vi "Finish.vi"   [LabVIEW 2015]
doc: "This VI is called just before exiting. It is expected to close I/O refnum, save collected data, etc."
uses:
  <vilib>/Rock Robotics/WPI/Utilities/WPI_GetSetVariantRefNum.vi
types:
  T1 = typedef "WPI_RobotDriveDevRef.ctl" = cluster{"DevStatus":errorcluster, "Motors[]":T2[], "Square Inputs":bool, "Max Output":dbl}
  T2 = typedef "WPI_MotorControlDeviceRef.ctl" = cluster{"DeviceStatus":errorcluster, "Type":T3, "PWM":cluster{"PWM Channel":T4, "DeadBand":T5}, "CAN":cluster{"Device Number":u8, "Control Mode":T6, "Semaphore":T7, "Max Vout":dbl, "TalonSRX Control Mode":T8}, "Invert":bool}
  T3 = typedef "WPI_MotorControlType.ctl" = enum16{"PWM", "CAN", "CANTalonSRX"}
  T4 = typedef "FPGA_DIOPWMChannel.ctl" = enum8{"PWM 0", "PWM 1", "PWM 2", "PWM 3", "PWM 4", "PWM 5", "PWM 6", "PWM 7", "PWM 8", "PWM 9", "PWM MXP 0", "PWM MXP 1", "PWM MXP 2", "PWM MXP 3", "PWM MXP 4", "PWM MXP 5", "PWM MXP 6", "PWM MXP 7", "PWM MXP 8", "PWM MXP 9", "Invalid"}
  T5 = typedef "WPI_PWMDeadband.ctl" = cluster{"Name":string, "maxPositivePwm":i32, "minPositivePwm":i32, "centerPwm":i32, "maxNegativePwm":i32, "minNegativePwm":i32, "angularRange":u16}
  T6 = typedef "WPI_CANJaguar_ControlMode.ctl" = enum8{"Percent VBus", "Current", "Speed", "Position", "Voltage"}
  T7 = typedef "Semaphore RefNum" = refnum<k1>
  T8 = typedef "WPI_CANTalonSRX_APIControlMode.ctl" = enum8{"Percent VBus", "Speed", "Position", "Slave", "Unchanged / Invalid", "Voltage Compensation", "Current", "Motion Profile"}
  T9 = typedef "WPI_SerialPortRef.ctl" = cluster{"DevStatus":errorcluster, "Serial Port Name":refnum<visa-resource-name>}
  T10 = typedef "WPI_SolenoidDevRef.ctl" = cluster{"DevStatus":errorcluster, "Pneumatics Control Module":u8, "Forward Solenoid Channel":T11, "Reverse Solenoid Channel":T11}
  T11 = typedef "WPI_SolenoidChannel.ctl" = enum8{"Solenoid 0", "Solenoid 1", "Solenoid 2", "Solenoid 3", "Solenoid 4", "Solenoid 5", "Solenoid 6", "Solenoid 7", "Invalid"}
  T12 = typedef "WPI_EncoderDevRef.ctl" = cluster{"DevStatus":errorcluster, "EncoderIndex":T13, "CounterIndex":T14, "DistancePerCount":dbl, "Decoding Type":T15}
  T13 = typedef "FPGA_EncoderIdx.ctl" = enum8{"Enc 0", "Enc 1", "Enc 2", "Enc 3", "Enc 4", "Enc 5", "Enc 6", "Enc 7", "Invalid"}
  T14 = typedef "FPGA_CounterCtrSystemIndex.ctl" = enum8{"Ctr 0", "Ctr 1", "Ctr 2", "Ctr 3", "Ctr 4", "Ctr 5", "Ctr 6", "Ctr 7", "Invalid"}
  T15 = typedef "WPI_EncoderType.ctl" = enum16{"1x", "2x", "4x"}
  T16 = typedef "WPI_JoystickDevRef.ctl" = cluster{"Device":T17}
  T17 = typedef "WPI_JoystickDeviceEnum.ctl" = enum16{"USB 0", "USB 1", "USB 2", "USB 3", "USB 4", "USB 5"}
  T18 = typedef "WPI_DigitalInputDevRef.ctl" = cluster{"DevStatus":errorcluster, "DIO Channel":T19}
  T19 = typedef "FPGA_DIOChannel.ctl" = enum8{"DIO 0", "DIO 1", "DIO 2", "DIO 3", "DIO 4", "DIO 5", "DIO 6", "DIO 7", "DIO 8", "DIO 9", "DIO MXP 0", "DIO MXP 1", "DIO MXP 2", "DIO MXP 3", "DIO MXP 4", "DIO MXP 5", "DIO MXP 6", "DIO MXP 7", "DIO MXP 8", "DIO MXP 9", "DIO MXP 10", "DIO MXP 11", "DIO MXP 12", "DIO MXP 13", "DIO MXP 14", "DIO MXP 15", "Invalid"}
  T20 = typedef "WPI_PotentiometerDevRef.ctl" = cluster{"DevStatus":errorcluster, "Analog Channel":T21, "Invert Output":bool}
  T21 = typedef "FPGA_AIChannel.ctl" = enum8{"AI 0", "AI 1", "AI 2", "AI 3", "AI MXP 0", "AI MXP 1", "AI MXP 2", "AI MXP 3", "Invalid"}
  T22 = typedef "WPI_GyroDevRef.ctl" = cluster{"DevStatus":errorcluster, "Analog Channel":T21, "Offset":dbl, "Gain (VoltsPerDegree/Second)":dbl, "Gyro Type":enum16{"Analog", "XRS450"}, "Handle":i32, "SPI Bus":T23, "Device Found":bool, "Sample Rate":dbl, "Calibrate On Open":bool}
  T23 = typedef "spi_bus.ctl" = enum16{"SPI On-Board, CS0", "SPI On-Board, CS1", "SPI On-Board, CS2", "SPI On-Board, CS3", "SPI MXP", "Invalid"}
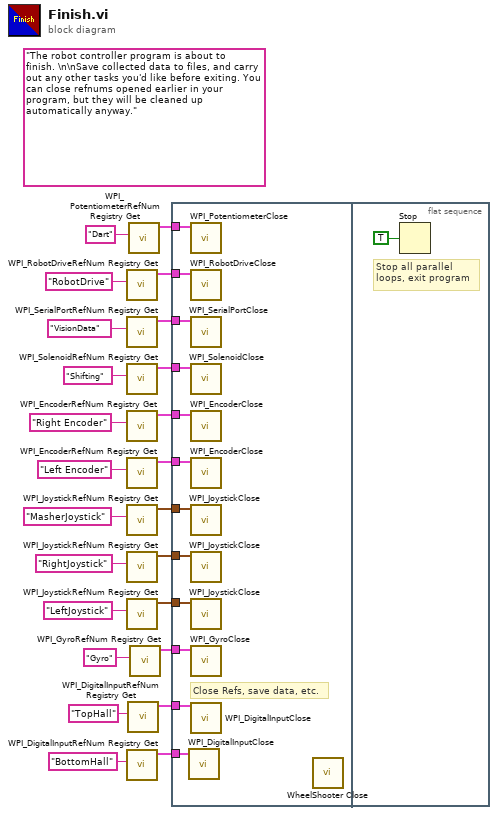
[diagram p0: block diagram]
diagram:
  (unwired) "The robot controller program is about to finish. \n\nSave collected data to files, and carry out any other tasks you'd like before exiting. You can close refnums opened earlier in your program, but they will be cleaned up automatically anyway."
  n1 = call <vilib>:"WPI_RobotDriveRefNum Registry Get.vi"("refnum name"="RobotDrive") -> ("RobotDriveDevRef"=w8:T1)  [unwired: 9 in, 1 out]
  n2 = call <vilib>:"WPI_SerialPortRefNum Registry Get.vi"("refnum name"="VisionData") -> ("SerialPortRef"=w10:T9)  [unwired: 9 in, 1 out]
  n3 = call <vilib>:"WPI_SolenoidRefNum Registry Get.vi"("refnum name"="Shifting") -> ("SolenoidDevRef"=w16:T10)  [unwired: 9 in, 1 out]
  n4 = call <vilib>:"WPI_EncoderRefNum Registry Get.vi"("refnum name"="Right Encoder") -> ("EncoderDevRef"=w17:T12)  [unwired: 9 in, 1 out]
  n5 = call <vilib>:"WPI_EncoderRefNum Registry Get.vi"("refnum name"="Left Encoder") -> ("EncoderDevRef"=w18:T12)  [unwired: 9 in, 1 out]
  n6 = call <vilib>:"WPI_JoystickRefNum Registry Get.vi"("refnum name"="MasherJoystick") -> ("JoystickDevRef"=w19:T16)  [unwired: 1 in, 9 out]
  n7 = call <vilib>:"WPI_JoystickRefNum Registry Get.vi"("refnum name"="RightJoystick") -> ("JoystickDevRef"=w20:T16)  [unwired: 1 in, 9 out]
  n8 = call <vilib>:"WPI_JoystickRefNum Registry Get.vi"("refnum name"="LeftJoystick") -> ("JoystickDevRef"=w23:T16)  [unwired: 1 in, 9 out]
  n9 = call <vilib>:"WPI_DigitalInputRefNum Registry Get.vi"("refnum name"="BottomHall") -> ("DigitalInputDevRef"=w4:T18)  [unwired: 9 in, 1 out]
  n10 = call <vilib>:"WPI_DigitalInputRefNum Registry Get.vi"("refnum name"="TopHall") -> ("DigitalInputDevRef"=w3:T18)  [unwired: 9 in, 1 out]
  n11 = call <vilib>:"WPI_PotentiometerRefNum Registry Get.vi"("refnum name"="Dart") -> ("PotDevRef"=w5:T20)  [unwired: 9 in, 1 out]
  n12 = call <vilib>:"WPI_GyroRefNum Registry Get.vi"("refnum name"="Gyro") -> ("GyroDevRef"=w15:T22)  [unwired: 9 in, 1 out]
  n13 = flat-sequence {
    tunnel: w23 -> [w36]
    tunnel: w20 -> [w35]
    tunnel: w19 -> [w34]
    tunnel: w18 -> [w33]
    tunnel: w17 -> [w32]
    tunnel: w16 -> [w31]
    tunnel: w15 -> [w30]
    tunnel: w10 -> [w29]
    tunnel: w8 -> [w28]
    tunnel: w5 -> [w27]
    tunnel: w4 -> [w26]
    tunnel: w3 -> [w25]
    frame #0 {
      # "Close Refs, save data, etc."
      n14 = call <vilib>:"WPI_DigitalInputClose.vi"("DigitalInputDevRef"=w26) -> ()  [unwired: 10 in, 1 out]
      n15 = call <vilib>:"WPI_PotentiometerClose.vi"("PotDevRef"=w27) -> ()  [unwired: 10 in, 1 out]
      n16 = call <vilib>:"WPI_RobotDriveClose.vi"("RobotDriveDevRef"=w28) -> ()  [unwired: 10 in, 1 out]
      n17 = call <vilib>:"WPI_SerialPortClose.vi"("SerialPortRef"=w29) -> ()  [unwired: 10 in, 1 out]
      n18 = call <vilib>:"WPI_SolenoidClose.vi"("SolenoidDevRef"=w31) -> ()  [unwired: 10 in, 1 out]
      n19 = call <vilib>:"WPI_EncoderClose.vi"("EncoderDevRef"=w32) -> ()  [unwired: 10 in, 1 out]
      n20 = call <vilib>:"WPI_EncoderClose.vi"("EncoderDevRef"=w33) -> ()  [unwired: 10 in, 1 out]
      n21 = call <vilib>:"WPI_JoystickClose.vi"("JoystickDevRef"=w34) -> ()  [unwired: 11 out]
      n22 = call <vilib>:"WPI_JoystickClose.vi"("JoystickDevRef"=w35) -> ()  [unwired: 11 out]
      n23 = call <vilib>:"WPI_JoystickClose.vi"("JoystickDevRef"=w36) -> ()  [unwired: 11 out]
      n24 = call <vilib>:"WPI_GyroClose.vi"("GyroDevRef"=w30) -> ()  [unwired: 10 in, 1 out]
      n25 = call <vilib>:"WPI_DigitalInputClose.vi"("DigitalInputDevRef"=w25) -> ()  [unwired: 10 in, 1 out]
      n26 = call "WheelShooter Close.vi"() -> ()  [unwired: 11 in, 1 out]
    }
    frame #1 {
      # "Stop all parallel\nloops, exit program"
      n27 = Stop(stop? (T)=TRUE ("Quit")) -> ()
    }
  }
